vi "Set Quiet Mode Functional Global.vi"(8 "Error In":errorcluster) -> (0 "Error Out":errorcluster)   [LabVIEW 2012, in "OpenCLV x64.lvlib"]
doc: "Halts the pop-ups when an error occurs. Error messages are still logged, but the option to continue, quit, or information about the error is not availible until the Error Log is viewed.\n\nThe pop-ups can be enabled by calling Verbose Mode, which can be found on the same polymorphic VI."
uses:
  OpenCLV x64.lvlib
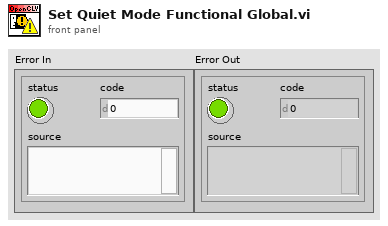
[diagram p1: front panel]
types:
  T1 = enum16{"Initialize", "Add Error", "View Error Log", "Save Error Log", "Set Verbose Mode", "Set Quite Mode"}
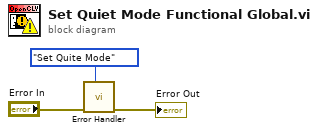
[diagram p0: block diagram]
diagram:
  n1 = call "Error Handler.vi"("Error Handler States"=T1."Set Quite Mode", "Error In"="Error In") -> ("Error Out"=→"Error Out":errorcluster)  [unwired: 9 in]
